vi "3d array testMOD1.vi"() -> ()   [LabVIEW 2011]
panel:
  in  "Stop Button":bool
  out "Intensity Slice":sgl[][](array[numeric])
  out "Array 3D":sgl[][][](array[numeric])
  in  "XY Plot Depth":u16(ring) items=["0", "1", "2", "3", "4"]
  in  "Plot":u16(ring) items=["XY", "X cross", "Y cross"]
  out "Intensity Graph":sgl[][](graph)
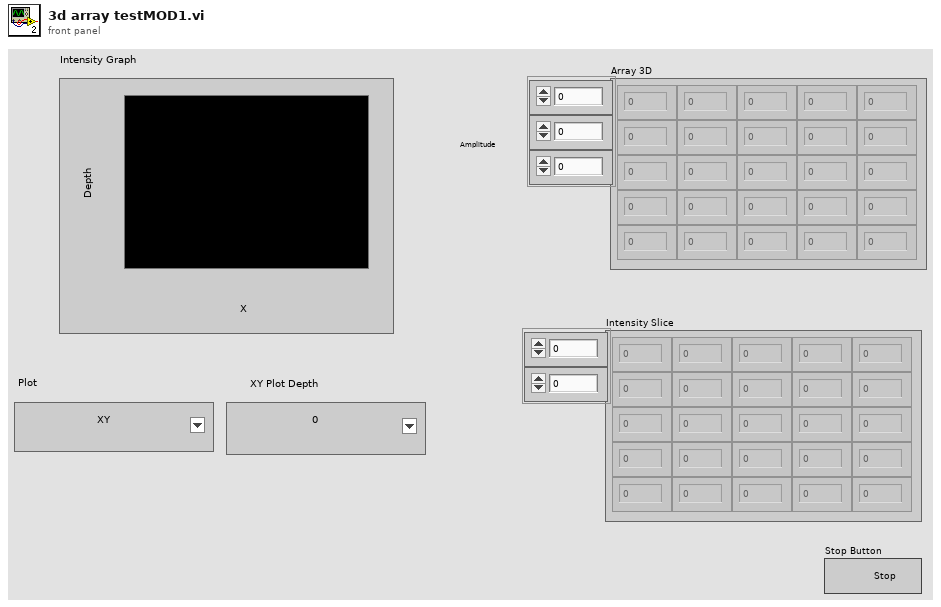
[diagram p1: front panel]
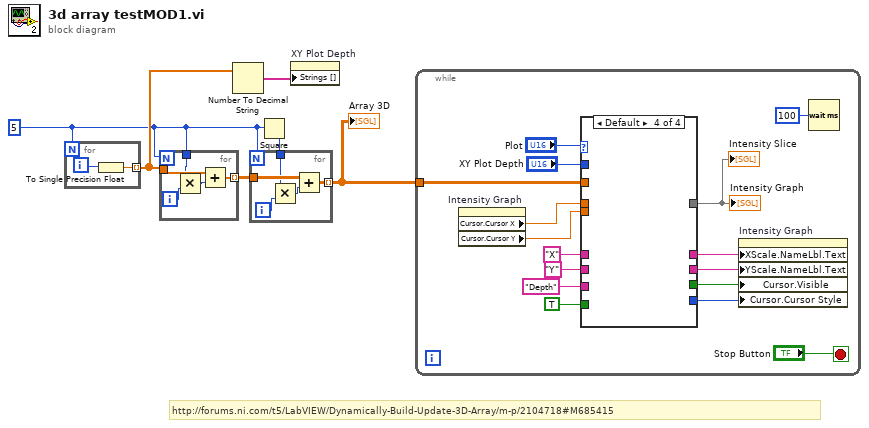
[diagram p0: block diagram]
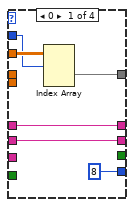
[diagram p2: hidden frame]
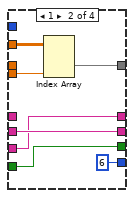
[diagram p3: hidden frame]
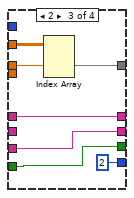
[diagram p4: hidden frame]
diagram:
  w2 = 5
  # "http://forums.ni.com/t5/LabVIEW/Dynamically-Build-Update-3D-Array/m-p/2104718#M685415"
  n1 = for {
    N: w2 -> [_]
    tunnel: [w8] -> w5 mode=indexing
    i -> [w7]
    n2 = To Single Precision Float(number=w7) -> (single precision float=w8:sgl)
  }
  n3 = for {
    N: w2 -> [_]
    tunnel: [w12] -> w4 mode=indexing
    tunnel: w5 -> [w13]
    tunnel: w2 -> [w9]
    i -> [w11]
    n4 = Multiply(x=w9, y=w11) -> (x*y=w10:i32)
    n5 = Add(x=w13, y=w10) -> (x+y=w12:sgl[])
  }
  n6 = Number To Decimal String(number=w5) -> (decimal integer string=w6:string[])  [unwired: 1 in]
  n7 = Square(x=w2) -> (x^2=w1:i32)
  n8 = for {
    N: w2 -> [_]
    tunnel: w4 -> [w18]
    tunnel: [w17] -> w3 mode=indexing
    tunnel: w1 -> [w15]
    i -> [w16]
    n9 = Multiply(x=w15, y=w16) -> (x*y=w14:i32)
    n10 = Add(x=w18, y=w14) -> (x+y=w17:sgl[][])
  }
  "Array 3D" <- w3
  n11 = property on="XY Plot Depth" class="Ring (strict)"("Strings []"=w6) -> ()  [unwired: 2 in, 2 out]
  n12 = while {
    tunnel: w3 -> [w25]
    stop <- "Stop Button" stop-if-true
    n13 = property on="Intensity Graph" class="IntGraph (strict)"() -> ("Cursor.Cursor X"=w31:dbl, "Cursor.Cursor Y"=w30:dbl)  [unwired: 2 in, 2 out]
    n14 = case shown="Default" "Plot" {
      tunnel: w25 -> [w40 w47 w54 _]
      tunnel: [w39 w46 w53 _] -> w24
      tunnel: "XY Plot Depth" -> [w36 _ _ _]
      tunnel: [w38 w44 w50 _] -> w32
      tunnel: w31 -> [_ _ w51 _]
      tunnel: w30 -> [_ w43 _ _]
      tunnel: [w37 w45 w52 _] -> w29
      tunnel: "X" ("X Scale.Name Label.Text") -> [w38 _ w50 _]
      tunnel: "Y" ("X Scale.Name Label.Text") -> [w37 w45 _ _]
      tunnel: "Depth" ("Y Scale.Name Label.Text") -> [_ w44 w52 _]
      tunnel: [u8 8 ("Cursor.Cursor Style") u8 6 ("Cursor.Cursor Style") u8 2 ("Cursor.Cursor Style") _] -> w21
      tunnel: [_ w41 w48 _] -> w20
      tunnel: TRUE -> [_ w41 w48 _]
      frame 0 {
        n15 = Index Array(array=w40, index (dim 0)=w36) -> (element=w39:sgl[][])  [unwired: 2 in]
      }
      frame 1 {
        n16 = Index Array(array=w47, index (dim 2)=w43) -> (element=w46:sgl[][])  [unwired: 2 in]
      }
      frame 2 {
        n17 = Index Array(array=w54, index (dim 1)=w51) -> (element=w53:sgl[][])  [unwired: 2 in]
      }
      frame Default {
      }
    }
    "Intensity Graph" <- w24
    "Intensity Slice" <- w24
    n18 = property on="Intensity Graph" class="IntGraph (strict)"("XScale.NameLbl.Text"=w32, "YScale.NameLbl.Text"=w29, "Cursor.Visible"=w20, "Cursor.Cursor Style"=w21) -> ()  [unwired: 2 in, 2 out]
    n19 = Wait (ms)(milliseconds to wait=u32 100) -> ()  [unwired: 1 out]
  }
